vi "Parse Response JSON.vi"(8 "error in (no error)":errorcluster, 10 "Response JSON":string, 11 "RGetInputMute in":refnum<class "RGetInputMute.lvclass">) -> (0 "error out":errorcluster, 3 "RGetInputMute out":refnum<class "RGetInputMute.lvclass">)   [LabVIEW 2022 SP3, in "obs-websocket-lv.lvlib" / "RGetInputMute.lvclass"]
uses:
  RGetInputMute.lvclass
  RGetInputMute.lvclass/RGetInputMute.ctl
  <vilib>/IlluminatedG/lv-web-crypto/lv-json/JSON/JSON.lvlib
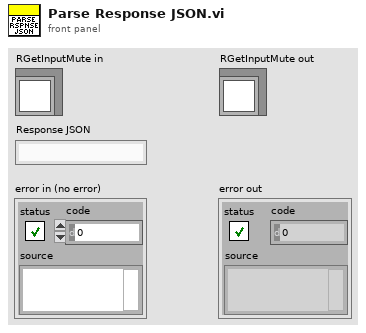
[diagram p1: front panel]
types:
  T1 = typedef "JSON.lvlib/JSON Item Type.ctl" = enum16{"unknown", "null", "Array", "Object", "String", "Number", "Boolean"}
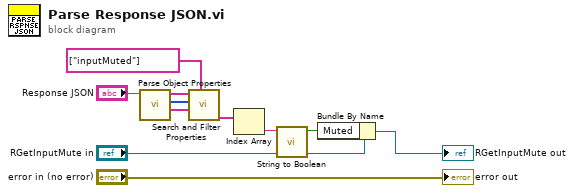
[diagram p0: block diagram]
diagram:
  n1 = call <vilib>:"Parse Object Properties.vi"("JSON String"="Response JSON") -> ("Values"=w7:string[], "Item Types"=w8:T1[], "Keys"=w9:string[])  [unwired: 7 in, 1 out]
  n2 = call <vilib>:"Search and Filter Properties.vi"("Search Keys"=string[] ["inputMuted"], "Values In"=w7, "Types In"=w8, "Keys In"=w9) -> ("Filtered Values"=w5:string[])  [unwired: 2 in, 5 out]
  n3 = Index Array(array=w5) -> (element=w4:string)  [unwired: 1 in]
  n4 = call <vilib>:"String to Boolean.vi"("Bool String"=w4) -> ("Boolean"=w3:bool)  [unwired: 10 in]
  n5 = Bundle By Name(cluster="RGetInputMute in", "Muted"=w3) -> (→"RGetInputMute out":refnum<class "RGetInputMute.lvclass">)
  "error out" <- "error in (no error)"
